vi "RunTest.vi"(8 "error in (no error)":errorcluster, 11 "Prueba06 in":refnum<class "Prueba06.lvclass">) -> (0 "error out":errorcluster, 2 "resultado":string, 3 "Prueba06 out":refnum<class "Prueba06.lvclass">)   [LabVIEW 2019, in "Prueba06.lvclass"]
uses:
  Prueba06.lvclass
  Prueba04/Control/Slide.ctl
  Control/MessageP06.ctl
  Control/EstadosP06.ctl
  Prueba06.lvclass/Prueba06.ctl
  <vilib>/Utility/miscctls.llb/LVRowAndColumnTypeDef.ctl
  ClusterGEN.ctl
  <vilib>/Utility/error.llb/DialogType.ctl
  QMH/Message Queue/Enqueue Message (Single).vi
  <vilib>/Utility/error.llb/Error Cluster From Error Code.vi
  <vilib>/ErrorRing/Error Ring.xnode
  Prueba/Prueba.lvclass
  Prueba04/Prueba04.lvclass
  QMH/User Event - Stop/User Event - Stop.lvlib
  QMH/Message Queue/Message Queue.lvlib
panel:
  out "Message":string
  out "voltaje11":dbl
  out "frecuencia11":dbl
  out "tipoPrueba":string
  out "filaSelecc":i32
  out "TablaVoltajes":string[](array[string])
  out "cumple_no_cumple":bool
  out "n° filas":i32
  out "ptoCentral":dbl=2.0 format="%#.1f"
  out "Vref":dbl
  in  "Tab":enum32{"Page 1", "Page 2"}(tab)
  out "voltaje1":dbl format="%.1f"
  out "RangoRef":string
  out "frecuencia1":dbl=140.0
  in  "guardar_Vref":bool
  out "nivelRef":dbl=95.0 format="%.1f"
  in  "generar1":bool
  in  "AjusteAmp":T1=50.0 caption="Ajuste de amplitud [mV]" scale=0.0..20000.0
  out "frecuencia1":dbl format="%.1f"
  in  "seguir":bool
  out "Pict Ring 3":u16(ring)
  out "Pict Ring 2":u16(ring)
  in  "generar2":bool caption="PruebaSup"
  in  "PruebaInf":bool caption="PruebaSup"
  in  "PruebaSup":bool
  in  "Tabla":string[][](table)
  in  "salir":bool
  out "cumple":bool
  out "no_cumple":bool
  out "voltaje2":dbl format="%.1f"
  out "frecuencia2":dbl format="%.1f"
  in  "cb_rangoRef":string(combo)="1000"
  out "RangoRef2":string
  # "Monitoreo"
  # "Frecuencia"
  # "Elección Señal de Referencia\nsegún marca y modelo de sonómetro"
  # "Hz"
  # "Voltaje"
  # "mV"
  # "Nivel Señal Referencia"
  # "Rango Referencia"
  # "Frecuencia"
  # "6. Linealidad de nivel en el rango de referencia. IEC 61672-3: 2006 Cláusula 14"
  # "Tabla Resultados"
  # "Rango [dBA]"
  # "Referencia [dBA]"
  # "Cumple"
  # "No Cumple"
  # "6. Linealidad de nivel en el rango de referencia. IEC 61672-3: 2006 Cláusula 14"
  # "Monitoreo"
  # "Frecuencia"
  # "Hz"
  # "Voltaje"
  # "mV"
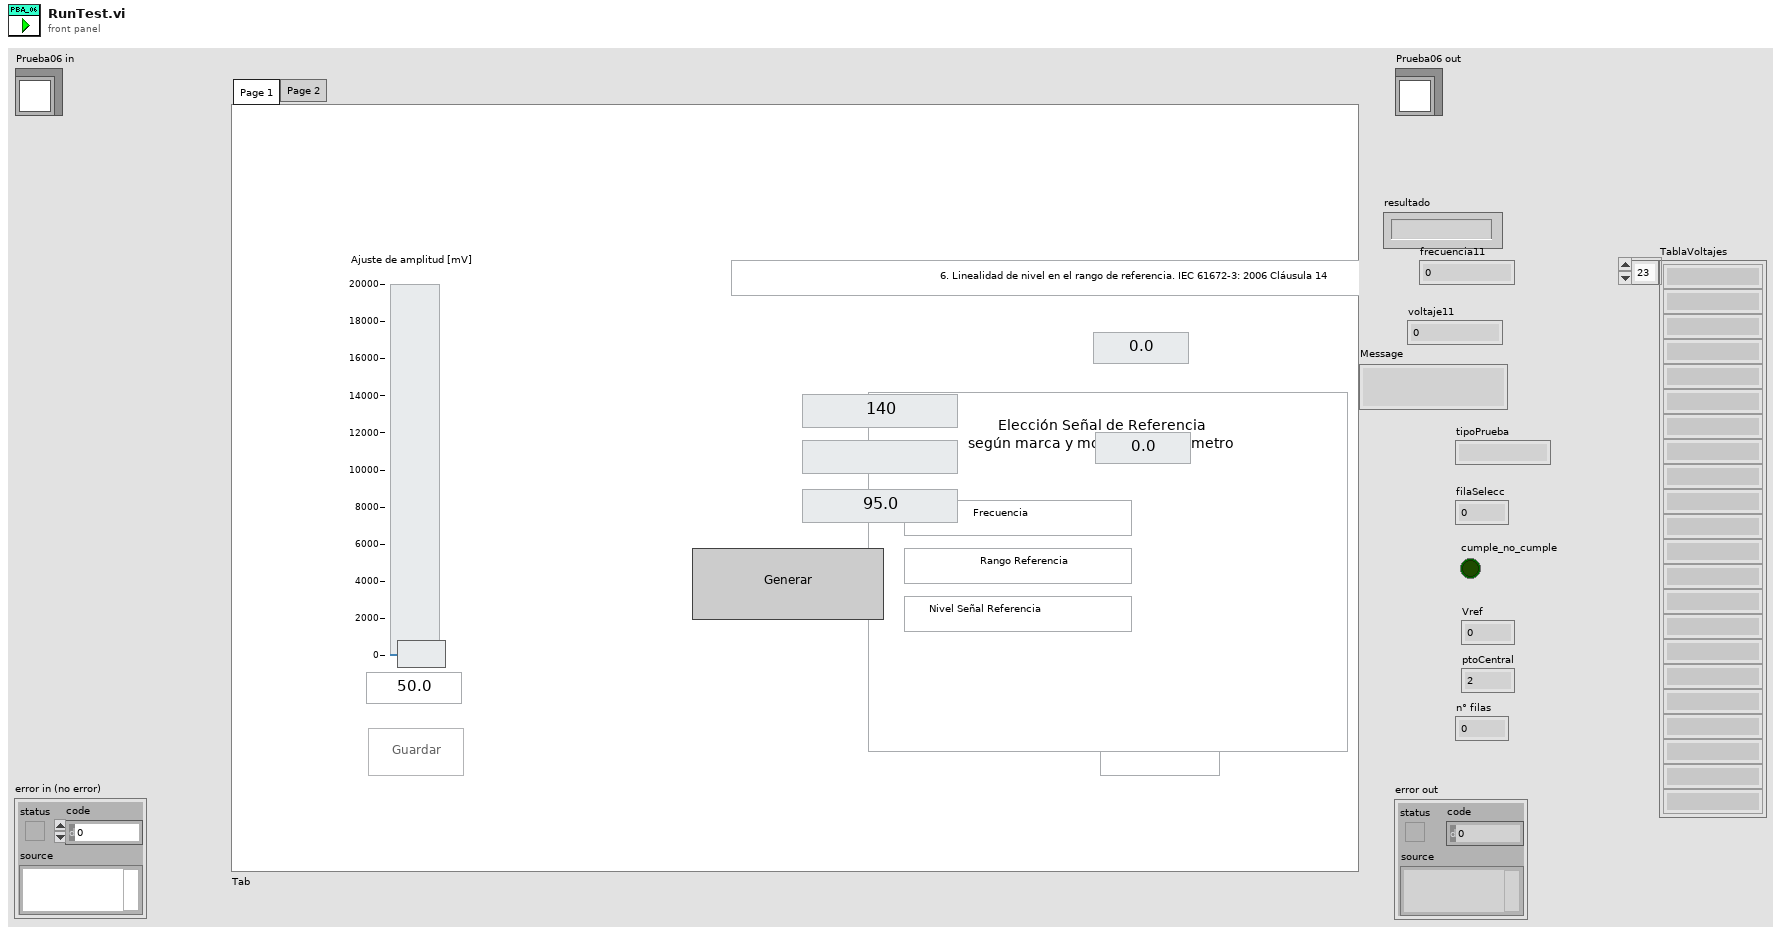
[diagram p1: front panel]
types:
  T1 = typedef "Prueba04.lvclass/Slide.ctl" = dbl
  T2 = typedef "LVRowAndColumnTypeDef.ctl" = cluster{"Row":i32, "Column":i32}
  T3 = typedef "Message Queue.lvlib/All Message Queues.ctl" = cluster{"MHL":refnum<queue>, "Inst_CNT90":refnum<queue>, "Inst_DS360":refnum<queue>, "Inst_Keithley2002":refnum<queue>, "Inst_DAQ":refnum<queue>, "BD":refnum<queue>, "Pistofono":refnum<queue>, "Nexus":refnum<queue>}
  T4 = enum8{"Enabled", "Disabled", "Disabled and Grayed Out"}
  T5 = typedef "Prueba06.lvclass/MessageP06.ctl" = cluster{"Estado":T6, "Data":variant}
  T6 = typedef "Prueba06.lvclass/EstadosP06.ctl" = enum16{"inicio", "LeerArchivoConfiguracion", "ConfirmarSalida", "DetieneInstrumentos", "InicializaInstrumento", "leerRango", "configuraRango", "calcularVref", "configuraTabla", "FrecAmp1", "FrecAmp2", "iniciarGEN", "monitoreo", "detenerGEN", "ajusteAmp", "guardaVerf", "creaVoltPrueba", "preguntaTipoPrueba", "guardarMediciones", "ingresaMediciones", "cumplimiento", "listo_evaluar", "evaluar", "final", "salir"}
  T7 = enum32{"Page 1", "Page 2", "Page 3", "Page 4", "Page 5", "Page 6", "Page 7"}
  T8 = typedef "Prueba06.lvclass/ClusterGEN.ctl" = cluster{"frec":dbl, "amp":dbl}
  T9 = cluster{"ControlName":string, "ControlReference":refnum<vi>}[]
  T10 = typedef "DialogType.ctl" = u16
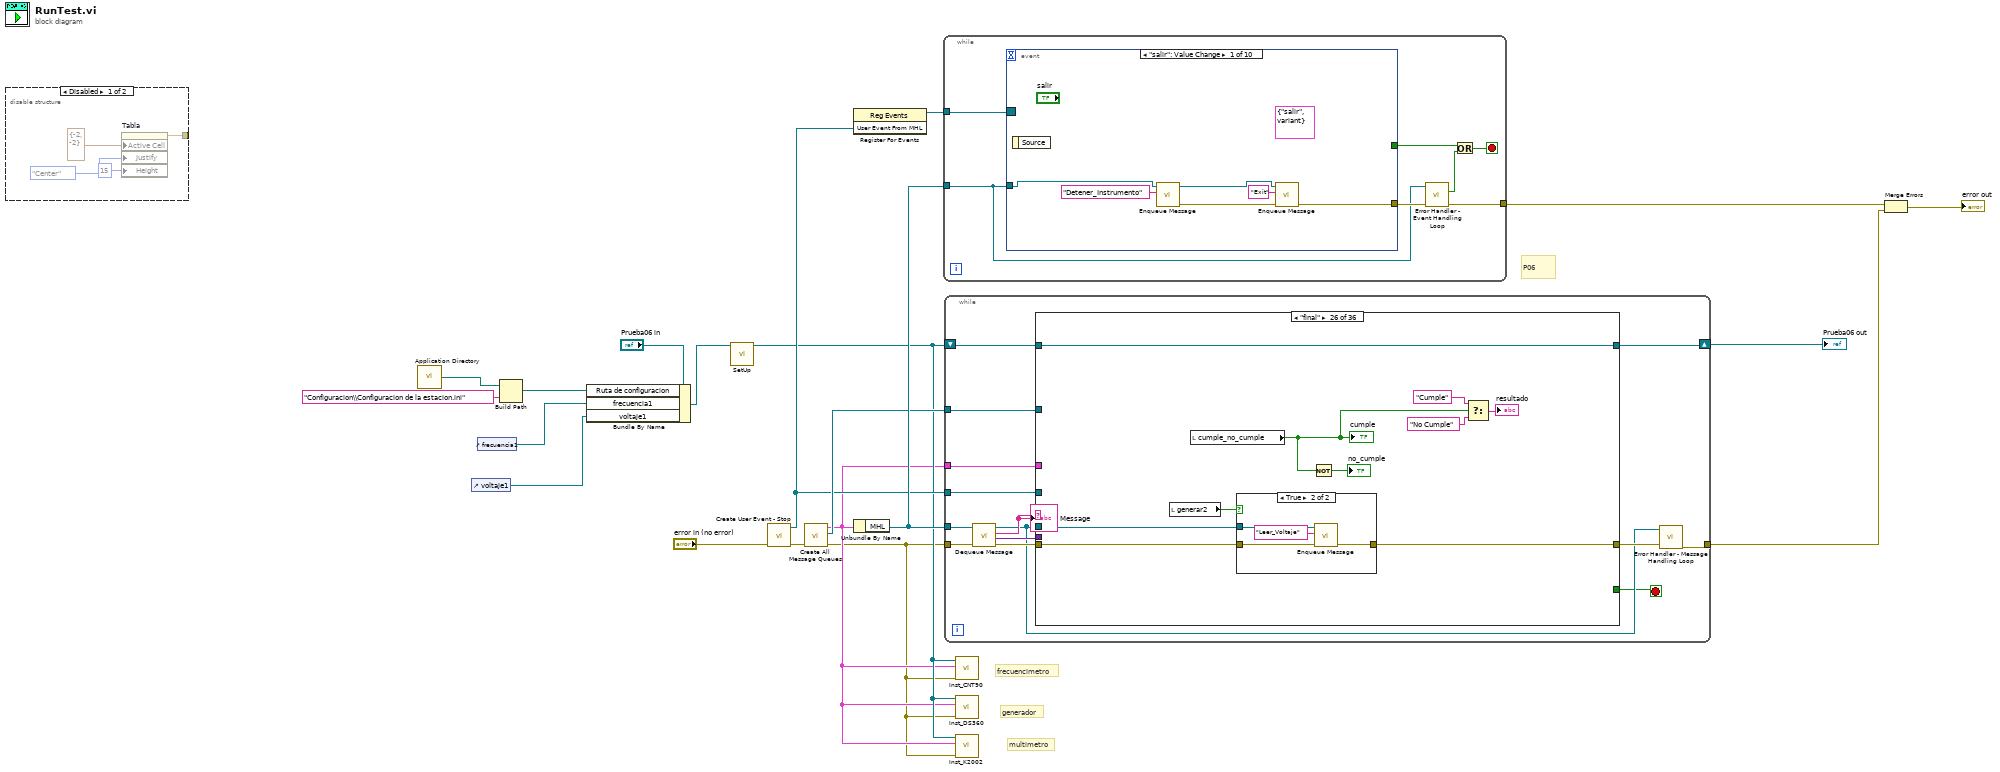
[diagram p0: block diagram]
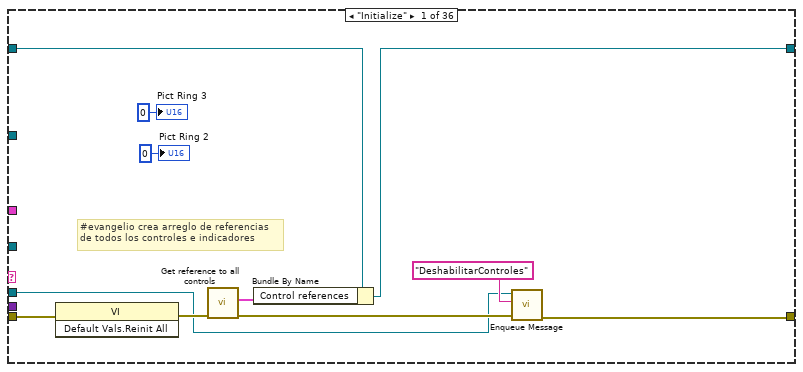
[diagram p3: hidden frame]
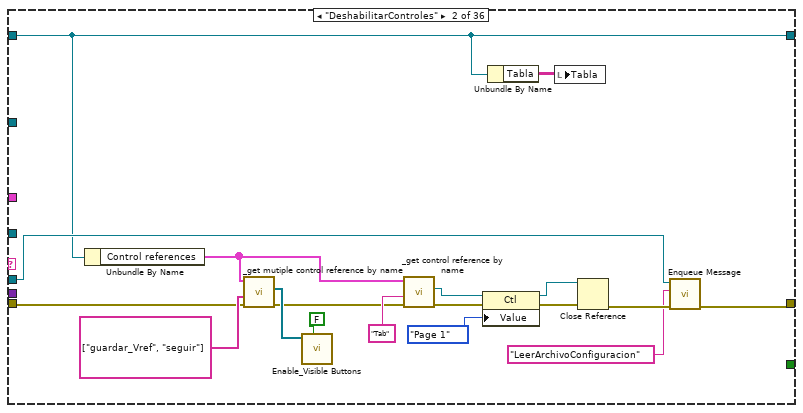
[diagram p4: hidden frame]
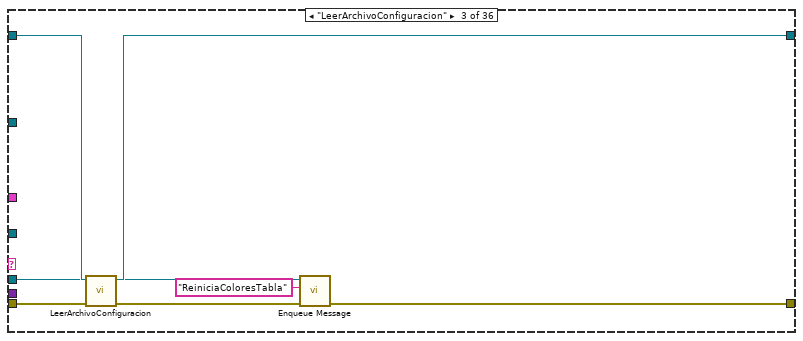
[diagram p5: hidden frame]
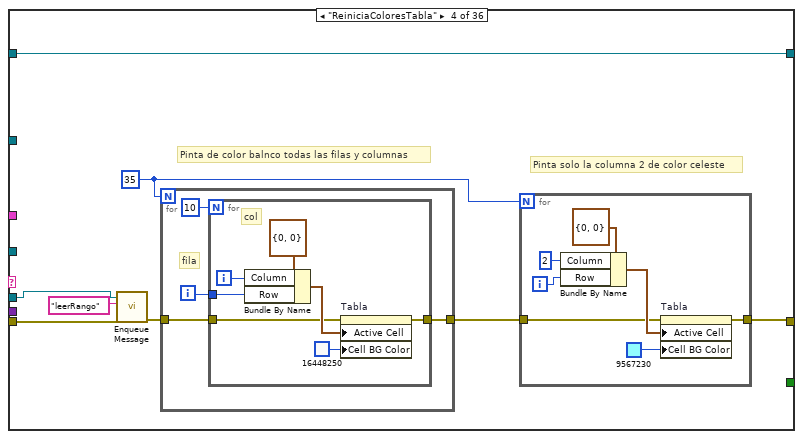
[diagram p6: hidden frame]
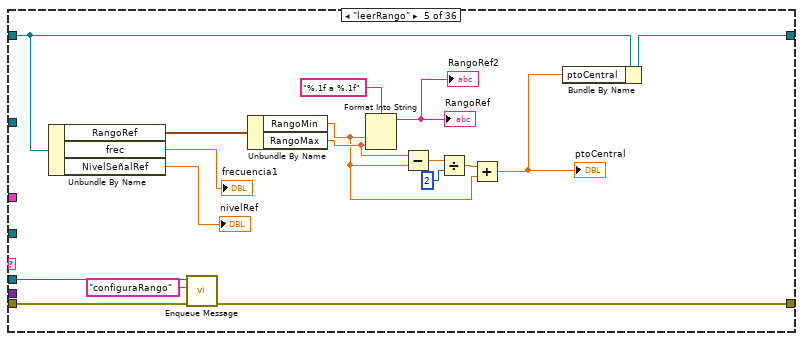
[diagram p7: hidden frame]
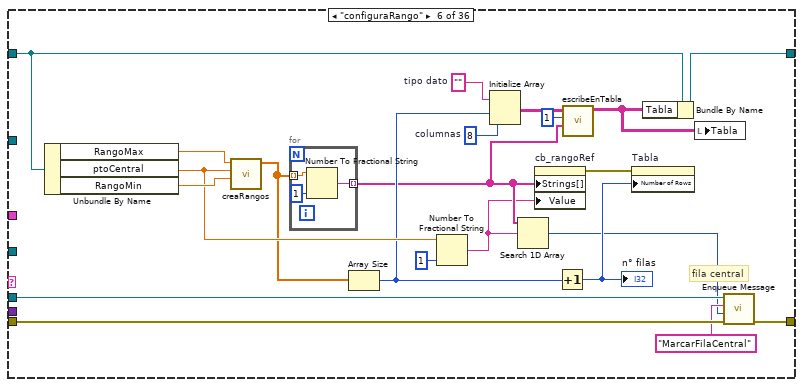
[diagram p8: hidden frame]
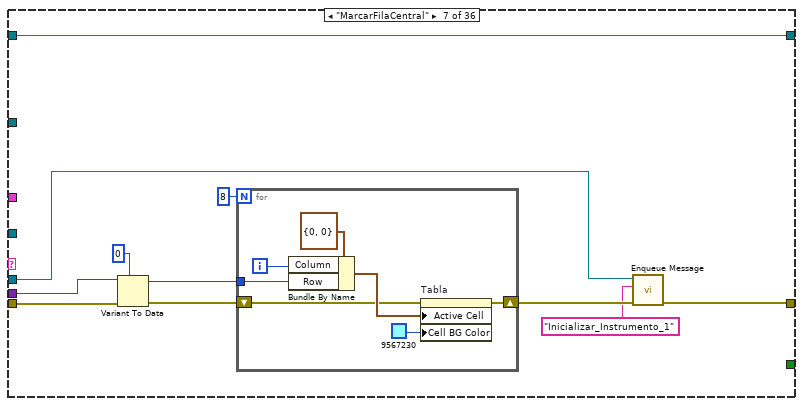
[diagram p9: hidden frame]
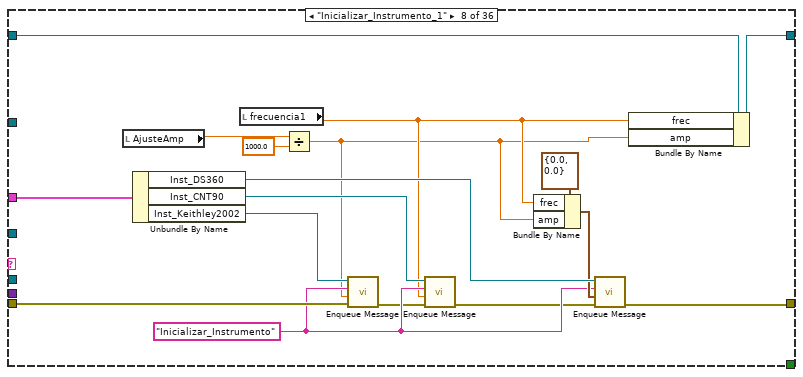
[diagram p10: hidden frame]
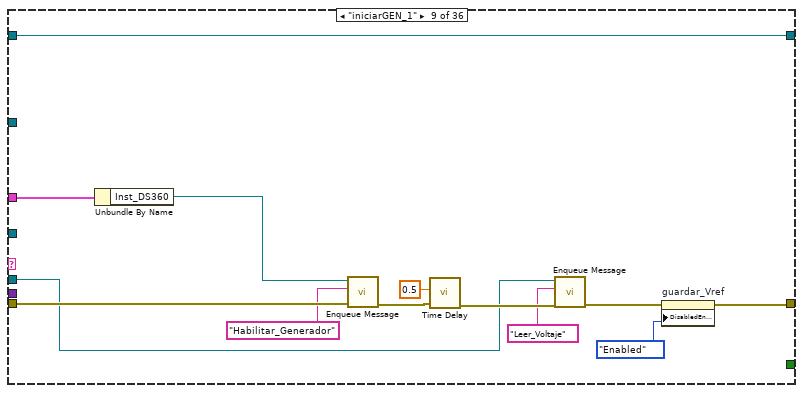
[diagram p11: hidden frame]
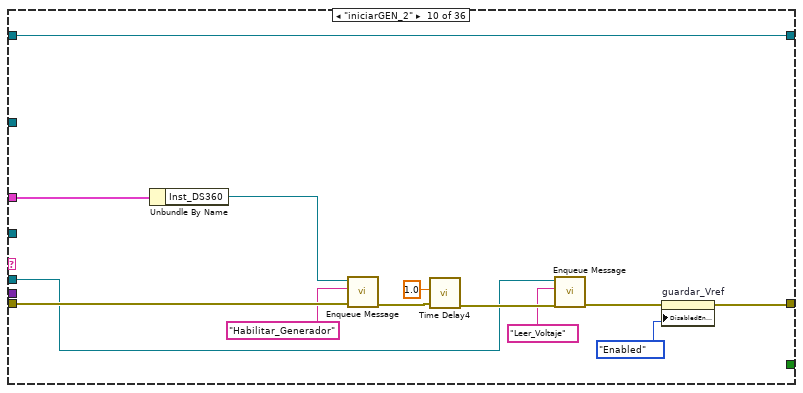
[diagram p12: hidden frame]
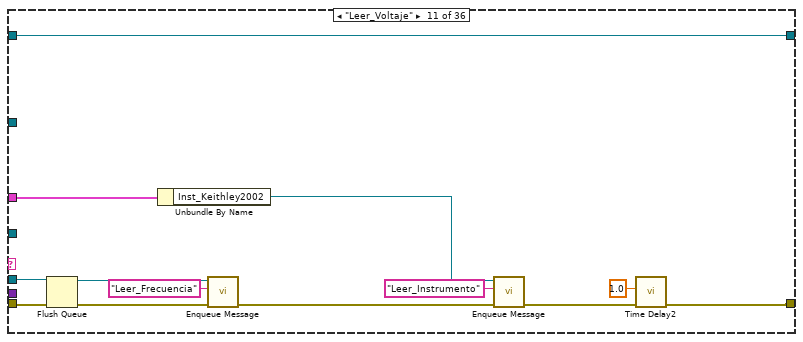
[diagram p13: hidden frame]
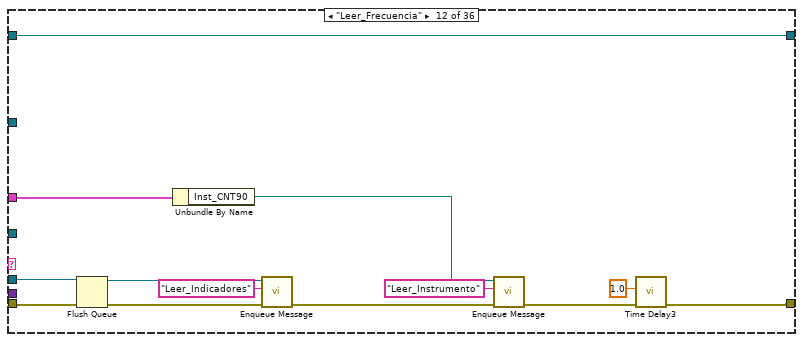
[diagram p14: hidden frame]
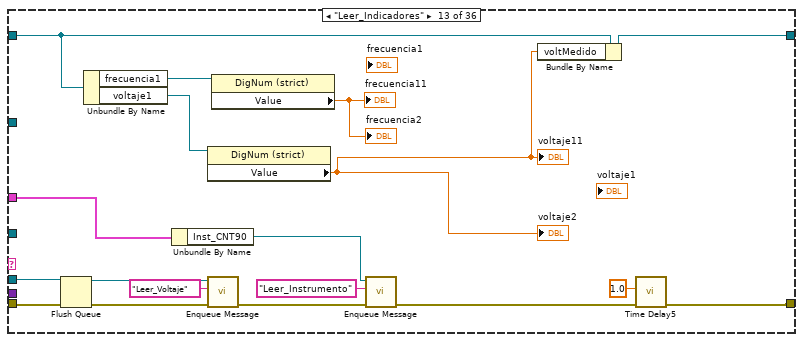
[diagram p15: hidden frame]
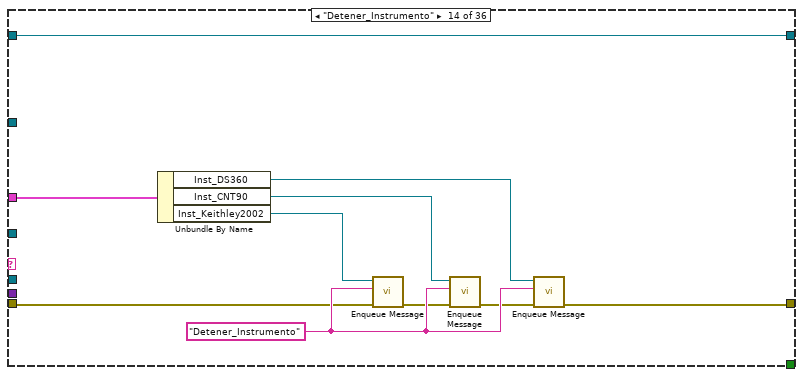
[diagram p16: hidden frame]
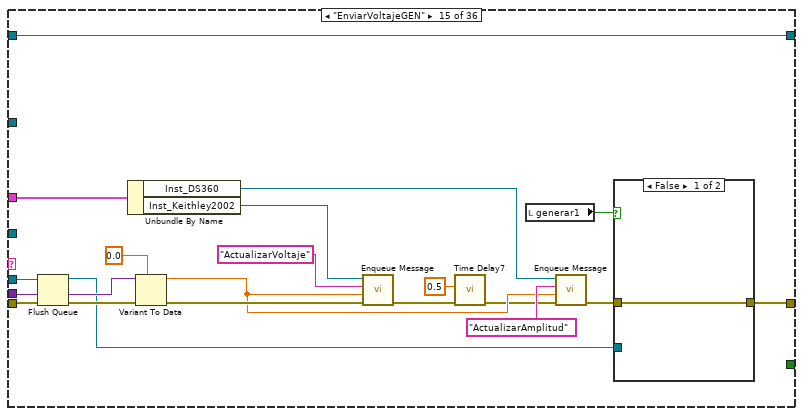
[diagram p17: hidden frame]
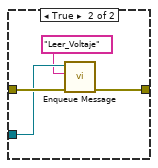
[diagram p18: hidden frame]
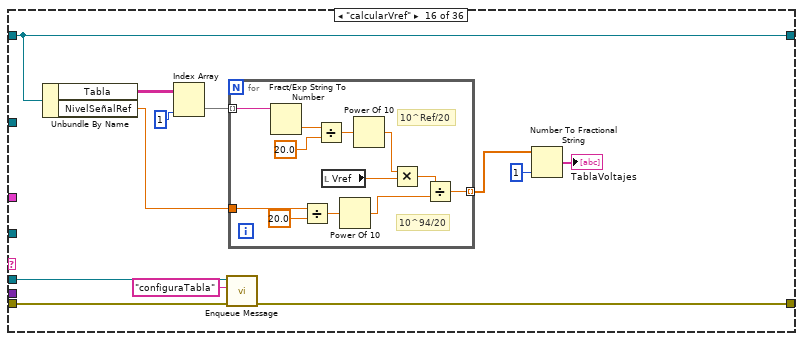
[diagram p19: hidden frame]
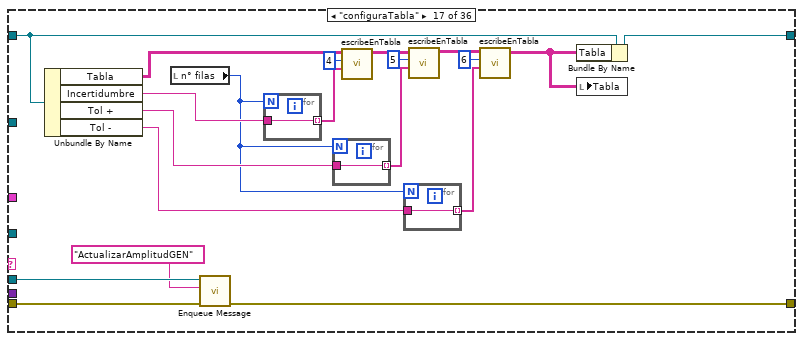
[diagram p20: hidden frame]
diagram:
  # "P06"
  # "multimetro"
  # "generador"
  # "frecuencimetro"
  n1 = disable-structure shown="Disabled" {
    disable-tunnel: [w23 _] -> _
    frame Disabled {
      n2 = property on="Tabla" class="Tbl (strict)"("Active Cell"=T2 {"Row"=-2, "Column"=-2} ("Active Cell:Active Cell"), "Justify"=enum16{"Left", "Center", "Right"}."Center" ("Active Cell:Cell Justification"), "Height"=u32 15 ("Active Cell:Cell Font:Size")) -> (error out=w23:errorcluster)  [unwired: 2 in, 1 out]
    }
    frame Enabled {
    }
  }
  n3 = call <vilib>:"Application Directory.vi"() -> ("Application Directory"=w15:path)
  n4 = control-ref of="voltaje1"() -> (w1:refnum<vi>)
  n5 = control-ref of="frecuencia1"() -> (w2:refnum<vi>)
  n6 = Build Path(base path=w15, name or relative path="Configuracion\\Configuracion de la estacion.ini") -> (appended path=w14:path)
  n7 = Bundle By Name(cluster="Prueba06 in", "Ruta de configuracion"=w14, "frecuencia1"=w2, "voltaje1"=w1) -> (w12:refnum<class "Prueba06.lvclass">)
  n8 = call-dynamic "SetUp.vi"("Prueba06 in"=w12) -> ("Prueba06 out"=w5:refnum<class "Prueba06.lvclass">)  [unwired: 9 in, 1 out]
  n9 = call "Create User Event - Stop.vi"("error in (no error)"="error in (no error)") -> ("error out"=w11:errorcluster, "User Event From MHL"=w7:refnum<user-event>)  [unwired: 9 in]
  n10 = call "Create All Message Queues.vi"("error in (no error)"=w11) -> ("error out"=w3:errorcluster, "PL Queues Array"=w8:refnum<queue>[], "All Message Queues out"=w4:T3)  [unwired: 8 in]
  n11 = register-events(w7) -> (reference out=w6:refnum<event-registration>)  [unwired: 2 in, 1 out]
  n12 = Unbundle By Name(w4) -> ("MHL"=w9:refnum<queue>)
  n13 = while {
    tunnel: w9 -> [w25]
    tunnel: [w29] -> w19
    tunnel: w6 -> [w27]
    stop <- w28 stop-if-true
    n14 = event shown="[0] \"salir\": Value Change" {
      selector: w27 -> [_ _ _ _ _ _ _ _ _ _]
      dyn-events: _ -> [_ _ _ _ _ _ _ _ _ _]
      timeout: _ -> [_ _ _ _ _ _ _ _ _ _]
      tunnel: w25 -> [w34 _ w45 w53 w60 w72 w78 w83 w88 w92]
      tunnel: [w37 _ _ w48 w55 w68 w79 w81 w87 w91] -> w30
      tunnel: [_ w38 _ _ _ _ _ _ _ _] -> w26
      event "salir": Value Change {
        (unwired) T5 {"Estado"=enum."salir", "Data"=variant} ("element")
        n15 = event-data() -> ()  [unwired: 1 in, 1 out]
        n16 = call-poly "Enqueue Message.vi"("Message"="Detener_Instrumento", "Message Queue"=w34) -> ("error out"=w32:errorcluster, "dup Message Queue"=w33:refnum<queue>)  [unwired: 8 in]
        n17 = call-poly "Enqueue Message.vi"("error in (no error)"=w32, "Message"="Exit", "Message Queue"=w33) -> ("error out"=w37:errorcluster)  [unwired: 7 in, 1 out]
      }
      event User Event {
        n18 = event-data() -> ("User Event"=w40:string, "Event Data"=w39:variant)  [unwired: 1 in]
        n19 = case shown="\"Exit EHL\"" w40 {
          tunnel: w39 -> [_ w42]
          tunnel: [_ w41] -> w38
          frame Default {
          }
          frame "Exit EHL" {
            # "#evangelio Termina\nla ejecucion del EHL"
            n20 = Variant To Data(type=TRUE, Variant=w42) -> (data=w41:bool)  [unwired: 1 in, 1 out]
          }
        }
      }
      event Panel Close? {
        w44 = TRUE
        n21 = event-data() -> ()  [unwired: 1 in, 1 out]
        n22 = call-poly "Enqueue Message.vi"("Priority Message? (F)"=w44, "Message"="Confirmar Salida", "Message Queue"=w45) -> ()  [unwired: 7 in, 2 out]
        n23 = event-data("Discard?"=w44) -> ()  [unwired: 1 in, 1 out]
      }
      event "generar1": Value Change {
        n24 = event-data() -> ("NewVal"=w52:bool)  [unwired: 1 in]
        n25 = Select(t="iniciarGEN_1", s=w52, f="detenerGEN") -> (s? t:f=w49:string)
        n26 = call-poly "Enqueue Message.vi"("Priority Message? (F)"=TRUE, "Message"=w49, "Message Queue"=w53) -> ("error out"=w48:errorcluster)  [unwired: 7 in, 1 out]
      }
      event "generar2": Value Change {
        n27 = event-data() -> ("NewVal"=w59:bool)  [unwired: 1 in]
        n28 = Select(t="preguntaTipoPrueba", s=w59, f="guardarMediciones") -> (s? t:f=w54:string)
        n29 = call-poly "Enqueue Message.vi"("Priority Message? (F)"=TRUE, "Message"=w54, "Message Queue"=w60) -> ("error out"=w61:errorcluster)  [unwired: 7 in, 1 out]
        n30 = case shown="\"preguntaTipoPrueba\", Default" w54 {
          tunnel: w61 -> [w64 w67]
          tunnel: [w63 w66] -> w55
          frame "preguntaTipoPrueba", Default {
            n31 = property on="cb_rangoRef" class="CmbBox"(error in=w64, "DisabledEnum"=T4."Disabled" ("Disabled")) -> (error out=w63:errorcluster)  [unwired: 1 in, 1 out]
          }
          frame "guardarMediciones" {
            n32 = property on="cb_rangoRef" class="CmbBox"(error in=w67, "DisabledEnum"=T4."Enabled" ("Disabled")) -> (error out=w66:errorcluster)  [unwired: 1 in, 1 out]
          }
        }
      }
      event "seguir": Value Change {
        n33 = event-data() -> ()  [unwired: 1 in, 1 out]
        n34 = call-poly "Enqueue Message.vi"("Message"="calcularVref", "Message Queue"=w72) -> ("error out"=w69:errorcluster)  [unwired: 8 in, 1 out]
        n35 = property on="Tab" class="TabCtl (strict)"(error in=w69, "Value"=enum32{"Page 1", "Page 2"}."Page 2" ("Tab")) -> (error out=w68:errorcluster)  [unwired: 1 in, 1 out]
      }
      event Value Change {
        (unwired) T5 {"Estado"=enum."FrecAmp1", "Data"=variant} ("element")
        n36 = event-data() -> ()  [unwired: 1 in, 1 out]
        n37 = Divide(x="AjusteAmp", y=T1 1000.0) -> (x/y=w74:T1)
        n38 = call-poly "Enqueue Message.vi"("Priority Message? (F)"=TRUE, "Message Data"=w74, "Message"="EnviarVoltajeGEN", "Message Queue"=w78) -> ("error out"=w79:errorcluster)  [unwired: 6 in, 1 out]
      }
      event "guardar_Vref": Value Change {
        (unwired) T5 {"Estado"=enum."guardaVerf", "Data"=variant} ("element")
        n39 = event-data() -> ()  [unwired: 1 in, 1 out]
        n40 = call-poly "Enqueue Message.vi"("Priority Message? (F)"=TRUE, "Message"="guardaVerf", "Message Queue"=w83) -> ("error out"=w81:errorcluster)  [unwired: 7 in, 1 out]
      }
      event "Tabla": Value Change {
        n41 = event-data() -> ("NewVal"=w85:string[][])  [unwired: 1 in]
        n42 = call-poly "Enqueue Message.vi"("Priority Message? (F)"=TRUE, "Message Data"=w85, "Message"="ingresaMediciones", "Message Queue"=w88) -> ("error out"=w87:errorcluster)  [unwired: 6 in, 1 out]
      }
      event "cb_rangoRef": Value Change {
        n43 = event-data() -> ()  [unwired: 1 in, 1 out]
        n44 = call-poly "Enqueue Message.vi"("Priority Message? (F)"=TRUE, "Message"="ActualizarAmplitudGEN", "Message Queue"=w92) -> ("error out"=w91:errorcluster)  [unwired: 7 in, 1 out]
      }
    }
    n45 = call "Error Handler - Event Handling Loop.vi"("error in (no error)"=w30, "Message Queue"=w25) -> ("dup error in"=w29:errorcluster, "Error?"=w31:bool)  [unwired: 7 in, 1 out]
    n46 = Or(x=w26, y=w31) -> (x .or. y?=w28:bool)
  }
  n47 = while {
    tunnel: w9 -> [w104]
    tunnel: w3 -> [w103]
    tunnel: [w93] -> w18
    shift-right: [w105] -> w20
    shift-left: w5 -> [w106]
    tunnel: w4 -> [w98]
    tunnel: w8 -> [w97]
    tunnel: w7 -> [w99]
    stop <- w94 stop-if-true
    n48 = call "Dequeue Message.vi"("error in (no error)"=w103, "Message Queue"=w104) -> ("error out"=w102:errorcluster, "Message Data"=w100:variant, "Message"=w101:string, "dup Message Queue"=w95:refnum<queue>)  [unwired: 6 in]
    "Message" <- w101
    n49 = case shown="\"final\"" w101 {
      selector: w101 -> [_ _ _ _ _ _ _ _ _ _ _ _ _ _ _ _ _ _ _ _ _ _ _ _ _ _ _ _ _ _ _ w639 _ _ _ w677]
      tunnel: [w110 w119 w140 w150 w184 w203 w221 w244 w258 w271 w284 w297 w300 w316 w345 w360 w387 w417 w442 w452 w465 w495 w510 w518 w543 w564 w574 w576 w590 w609 w623 w630 w655 w673 w675 w678] -> w105
      tunnel: w106 -> [w111 w119 w141 w150 w185 w205 w221 w245 w258 w271 w284 w297 w306 w316 w345 w360 w388 w418 w443 w452 w482 w506 w514 w518 w543 w564 w574 w581 w590 w609 w623 w631 w655 w673 w675 w678]
      tunnel: w100 -> [_ _ _ _ _ _ w219 _ _ _ _ _ _ _ w335 _ _ _ _ _ _ w499 _ _ _ _ w572 w578 _ _ _ _ _ w664 _ _]
      tunnel: w102 -> [w112 w121 w142 w148 w183 w197 w220 w243 w257 w270 w276 w289 w308 w319 w336 w358 w386 w416 w441 w448 w483 w508 w516 w525 w546 w562 w573 w580 w592 w611 w622 w640 w650 w667 w674 _]
      tunnel: [w109 w118 w137 w144 w174 w191 w213 w233 w253 w266 w275 w288 w307 w317 w328 w356 w377 w402 w433 w445 w462 w505 w513 w524 w544 w557 w571 w579 w591 w610 w619 w635 w648 w665 w674 w676] -> w96
      tunnel: [_ _ _ _ _ _ _ _ _ _ _ _ _ _ _ _ _ _ _ _ _ _ _ _ _ _ _ _ _ _ _ w636 _ _ _ _] -> w94
      tunnel: w95 -> [w113 w120 w138 w147 w173 w190 w212 _ w247 w260 w273 w286 w302 _ w331 w357 w376 _ _ w446 w479 w502 w512 w523 w545 w556 _ _ w583 w603 _ w634 w649 w666 _ _]
      tunnel: w99 -> [_ _ _ _ _ _ _ _ _ _ _ _ _ _ _ _ _ _ _ _ _ _ _ _ _ _ _ _ _ _ _ w637 _ _ _ _]
      tunnel: w98 -> [_ _ _ _ _ _ _ w229 w252 w265 w277 w290 w309 w318 w334 _ _ w401 w432 _ _ _ _ _ _ _ _ _ w593 w612 _ _ _ _ _ _]
      tunnel: w97 -> [_ _ _ _ _ _ _ _ _ _ _ _ _ _ _ _ _ _ _ _ _ _ _ _ _ _ _ _ _ _ _ w638 _ _ _ _]
      frame "Initialize" {
        # "#evangelio crea arreglo de referencias\nde todos los controles e indicadores"
        n50 = invoke class="VI" method="Default Vals.Reinit All"(error in=w112) -> (error out=w116:errorcluster)  [unwired: 2 in, 2 out]
        n51 = call "Get reference to all controls.vi"("error in (no error)"=w116) -> ("error out"=w114:errorcluster, "Control references"=w115:T9)  [unwired: 5 in]
        n52 = Bundle By Name(cluster=w111, "Control references"=w115) -> (w110:refnum<class "Prueba06.lvclass">)
        n53 = call-poly "Enqueue Message.vi"("error in (no error)"=w114, "Message"="DeshabilitarControles", "Message Queue"=w113) -> ("error out"=w109:errorcluster)  [unwired: 7 in, 1 out]
        "Pict Ring 2" <- u16 0 ("Pict Ring 2")
        "Pict Ring 3" <- u16 0 ("Pict Ring 3")
      }
      frame "DeshabilitarControles" {
        n54 = Unbundle By Name(w119) -> ("Control references"=w130:T9)
        n55 = call "_get mutiple control reference by name.vi"("error in (no error)"=w121, "Control names"=string[] ["guardar_Vref", "seguir"], "Control references"=w130) -> ("error out"=w127:errorcluster, "References"=w128:refnum<vi>[])  [unwired: 3 in]
        n56 = call "Enable_Visible Buttons.vi"("Enable? (T)"=FALSE, "Controls Ref Array"=w128) -> ()  [unwired: 10 in]
        n57 = call "_get control reference by name.vi"("error in (no error)"=w127, "Control name"="Tab" ("Message"), "Control references"=w130) -> ("error out"=w134:errorcluster, "Ctl Refnum"=w132:refnum<vi>)  [unwired: 3 in]
        n58 = property class="Ctl"(reference=w132, error in=w134, "Value"=T7."Page 1" ("Tab_Prueba04")) -> (reference out=w123:refnum<vi>, error out=w125:errorcluster)
        n59 = Unbundle By Name(w119) -> ("Tabla"=w135:string[][])
        n60 = local write "Tabla"(w135) -> ()
        n61 = Close Reference(reference=w123, error in (no error)=w125) -> (error out=w124:errorcluster)
        n62 = call-poly "Enqueue Message.vi"("error in (no error)"=w124, "Message"="LeerArchivoConfiguracion", "Message Queue"=w120) -> ("error out"=w118:errorcluster)  [unwired: 7 in, 1 out]
      }
      frame "LeerArchivoConfiguracion" {
        n63 = call "LeerArchivoConfiguracion.vi"("error in"=w142, "Prueba06 in"=w141) -> ("error out"=w139:errorcluster, "Prueba06 out"=w140:refnum<class "Prueba06.lvclass">)  [unwired: 8 in]
        n64 = call-poly "Enqueue Message.vi"("error in (no error)"=w139, "Message"="ReiniciaColoresTabla", "Message Queue"=w138) -> ("error out"=w137:errorcluster)  [unwired: 7 in, 1 out]
      }
      frame "ReiniciaColoresTabla" {
        w143 = 35
        # "Pinta solo la columna 2 de color celeste"
        # "Pinta de color balnco todas las filas y columnas"
        n65 = call-poly "Enqueue Message.vi"("error in (no error)"=w148, "Message"="leerRango", "Message Queue"=w147) -> ("error out"=w146:errorcluster)  [unwired: 7 in, 1 out]
        n66 = for {
          N: w143 -> [_]
          tunnel: w146 -> [w154]
          tunnel: [w153] -> w145
          i -> [w152]
          # "fila"
          n67 = for {
            N: 10 -> [_]
            tunnel: [w158] -> w153
            tunnel: w154 -> [w157]
            tunnel: w152 -> [w156]
            i -> [w155]
            # "col"
            n68 = Bundle By Name(cluster=T2 {"Row"=0, "Column"=0} ("Active Cell:Active Cell"), "Column"=w155, "Row"=w156) -> (w160:T2)
            n69 = property on="Tabla" class="Tbl (strict)"(error in=w157, "Active Cell"=w160, "Cell BG Color"=u32 16448250) -> (error out=w158:errorcluster)  [unwired: 1 in, 1 out]
          }
        }
        n70 = for {
          N: w143 -> [_]
          tunnel: [w164] -> w144
          tunnel: w145 -> [w162]
          i -> [w163]
          n71 = Bundle By Name(cluster=T2 {"Row"=0, "Column"=0} ("Active Cell:Active Cell"), "Column"=2, "Row"=w163) -> (w166:T2)
          n72 = property on="Tabla" class="Tbl (strict)"(error in=w162, "Active Cell"=w166, "Cell BG Color"=u32 9567230) -> (error out=w164:errorcluster)  [unwired: 1 in, 1 out]
        }
      }
      frame "leerRango" {
        n73 = Unbundle By Name(w185) -> ("RangoRef"=w182:cluster{"RangoMin":dbl, "RangoMax":dbl}, "frec"=→"frecuencia1":dbl, "NivelSeñalRef"=→"nivelRef":dbl)
        n74 = call-poly "Enqueue Message.vi"("error in (no error)"=w183, "Message"="configuraRango", "Message Queue"=w173) -> ("error out"=w174:errorcluster)  [unwired: 7 in, 1 out]
        n75 = Unbundle By Name(w182) -> ("RangoMin"=w175:dbl, "RangoMax"=w180:dbl)
        n76 = Format Into String(format string="%.1f a %.1f", w175, w180) -> (resulting string=→"RangoRef" →"RangoRef2":string)  [unwired: 2 in, 1 out]
        n77 = Subtract(x=w180, y=w175) -> (x-y=w177:dbl)
        n78 = Divide(x=w177, y=u32 2) -> (x/y=w178:dbl)
        n79 = Add(x=w178, y=w175) -> (x+y=w179:dbl)
        "ptoCentral" <- w179
        n80 = Bundle By Name(cluster=w185, "ptoCentral"=w179) -> (w184:refnum<class "Prueba06.lvclass">)
      }
      frame "configuraRango" {
        w196 = 8  # columnas
        w195 = ""  # tipo dato
        # "fila central"
        n81 = Unbundle By Name(w205) -> ("RangoMax"=w207:dbl, "ptoCentral"=w202:dbl, "RangoMin"=w206:dbl)
        n82 = call "creaRangos.vi"("RangoMin"=w206, "ptoCentral"=w202, "RangoMax"=w207) -> ("RangoCompleto"=w201:dbl[])  [unwired: 5 in, 3 out]
        n83 = for {
          tunnel: w201 -> [w210] mode=indexing
          tunnel: [w209] -> w188 mode=indexing
          n84 = Number To Fractional String(number=w210, precision (6)=i16 1) -> (F-format string=w209:string)  [unwired: 2 in]
        }
        n85 = Array Size(array=w201) -> (size(s)=w194:i32)
        n86 = Number To Fractional String(number=w202, precision (6)=i16 1) -> (F-format string=w187:string)  [unwired: 2 in]
        n87 = Initialize Array(w195, w194, w196) -> (w193:string[][])
        n88 = Search 1D Array(1D array=w188, element=w187) -> (index of element=w186:i32)  [unwired: 1 in]
        n89 = property on="cb_rangoRef" class="CmbBox"("Strings[]"=w188, "Value"=w187) -> (error out=w200:errorcluster)  [unwired: 2 in, 1 out]
        n90 = Increment(x=w194) -> (x+1=w199:i32)
        "n° filas" <- w199
        n91 = call "escribeEnTabla.vi"("parametros"=w188, "col"=1, "tabla in"=w193) -> ("tabla out"=w192:string[][])  [unwired: 8 in]
        n92 = property on="Tabla" class="Tbl (strict)"(error in=w200, "Number of Rows"=w199) -> ()  [unwired: 1 in, 2 out]
        n93 = Bundle By Name(cluster=w205, "Tabla"=w192) -> (w203:refnum<class "Prueba06.lvclass">)
        n94 = local write "Tabla"(w192) -> ()
        n95 = call-poly "Enqueue Message.vi"("error in (no error)"=w197, "Message Data"=w186, "Message"="MarcarFilaCentral", "Message Queue"=w190) -> ("error out"=w191:errorcluster)  [unwired: 6 in, 1 out]
      }
      frame "MarcarFilaCentral" {
        n96 = Variant To Data(error in=w220, type=0, Variant=w219) -> (data=w215:i32, error out=w217:errorcluster)
        n97 = for {
          N: 8 -> [_]
          tunnel: w215 -> [w223]
          shift-right: [w224] -> w216
          shift-left: w217 -> [w225]
          i -> [w222]
          n98 = Bundle By Name(cluster=T2 {"Row"=0, "Column"=0} ("Active Cell:Active Cell"), "Column"=w222, "Row"=w223) -> (w227:T2)
          n99 = property on="Tabla" class="Tbl (strict)"(error in=w225, "Active Cell"=w227, "Cell BG Color"=u32 9567230) -> (error out=w224:errorcluster)  [unwired: 1 in, 1 out]
        }
        n100 = call-poly "Enqueue Message.vi"("error in (no error)"=w216, "Message"="Inicializar_Instrumento_1", "Message Queue"=w212) -> ("error out"=w213:errorcluster)  [unwired: 7 in, 1 out]
      }
      frame "Inicializar_Instrumento_1" {
        w236 = "Inicializar_Instrumento" ("Message")
        n101 = local read "AjusteAmp"() -> (w242:T1)
        n102 = Unbundle By Name(w229) -> ("Inst_DS360"=w240:refnum<queue>, "Inst_CNT90"=w239:refnum<queue>, "Inst_Keithley2002"=w238:refnum<queue>)
        n103 = local read "frecuencia1"() -> (w231:dbl)
        n104 = Divide(x=w242, y=T1 1000.0) -> (x/y=w230:T1)
        n105 = call-poly "Enqueue Message.vi"("error in (no error)"=w243, "Message Data"=w230, "Message"=w236, "Message Queue"=w238) -> ("error out"=w235:errorcluster)  [unwired: 6 in, 1 out]
        n106 = call-poly "Enqueue Message.vi"("error in (no error)"=w235, "Message Data"=w231, "Message"=w236, "Message Queue"=w239) -> ("error out"=w234:errorcluster)  [unwired: 6 in, 1 out]
        n107 = Bundle By Name(cluster=T8 {"frec"=0.0, "amp"=0.0} ("clusterGEN"), "frec"=w231, "amp"=w230) -> (w237:T8)
        n108 = call-poly "Enqueue Message.vi"("error in (no error)"=w234, "Message Data"=w237, "Message"=w236, "Message Queue"=w240) -> ("error out"=w233:errorcluster)  [unwired: 6 in, 1 out]
        n109 = Bundle By Name(cluster=w245, "frec"=w231, "amp"=w230) -> (w244:refnum<class "Prueba06.lvclass">)
      }
      frame "iniciarGEN_1" {
        n110 = Unbundle By Name(w252) -> ("Inst_DS360"=w251:refnum<queue>)
        n111 = call-poly "Enqueue Message.vi"("error in (no error)"=w257, "Message"="Habilitar_Generador", "Message Queue"=w251) -> ("error out"=w249:errorcluster)  [unwired: 7 in, 1 out]
        n112 = call "Time Delay"("error in (no error)"=w249, "Delay Time (s)"=0.5) -> ("error out"=w248:errorcluster)  [unwired: 9 in]
        n113 = call-poly "Enqueue Message.vi"("error in (no error)"=w248, "Message"="Leer_Voltaje", "Message Queue"=w247) -> ("error out"=w254:errorcluster)  [unwired: 7 in, 1 out]
        n114 = property on="guardar_Vref" class="Bool"(error in=w254, "DisabledEnum"=T4."Enabled" ("Disabled")) -> (error out=w253:errorcluster)  [unwired: 1 in, 1 out]
      }
      frame "iniciarGEN_2" {
        n115 = Unbundle By Name(w265) -> ("Inst_DS360"=w264:refnum<queue>)
        n116 = call-poly "Enqueue Message.vi"("error in (no error)"=w270, "Message"="Habilitar_Generador", "Message Queue"=w264) -> ("error out"=w262:errorcluster)  [unwired: 7 in, 1 out]
        n117 = call "Time Delay4"("error in (no error)"=w262, "Delay Time (s)"=1.0) -> ("error out"=w261:errorcluster)  [unwired: 9 in]
        n118 = call-poly "Enqueue Message.vi"("error in (no error)"=w261, "Message"="Leer_Voltaje", "Message Queue"=w260) -> ("error out"=w267:errorcluster)  [unwired: 7 in, 1 out]
        n119 = property on="guardar_Vref" class="Bool"(error in=w267, "DisabledEnum"=T4."Enabled" ("Disabled")) -> (error out=w266:errorcluster)  [unwired: 1 in, 1 out]
      }
      frame "Leer_Voltaje" {
        n120 = Flush Queue(queue=w273, error in (no error)=w276) -> (queue out=w272:refnum<queue>, error out=w274:errorcluster)  [unwired: 1 out]
        n121 = Unbundle By Name(w277) -> ("Inst_Keithley2002"=w280:refnum<queue>)
        n122 = call-poly "Enqueue Message.vi"("error in (no error)"=w274, "Message"="Leer_Frecuencia", "Message Queue"=w272) -> ("error out"=w283:errorcluster)  [unwired: 7 in, 1 out]
        n123 = call-poly "Enqueue Message.vi"("error in (no error)"=w283, "Message"="Leer_Instrumento", "Message Queue"=w280) -> ("error out"=w281:errorcluster)  [unwired: 7 in, 1 out]
        n124 = call "Time Delay2"("error in (no error)"=w281, "Delay Time (s)"=1.0) -> ("error out"=w275:errorcluster)  [unwired: 9 in]
      }
      frame "Leer_Frecuencia" {
        n125 = Flush Queue(queue=w286, error in (no error)=w289) -> (queue out=w285:refnum<queue>, error out=w287:errorcluster)  [unwired: 1 out]
        n126 = Unbundle By Name(w290) -> ("Inst_CNT90"=w293:refnum<queue>)
        n127 = call-poly "Enqueue Message.vi"("error in (no error)"=w287, "Message"="Leer_Indicadores", "Message Queue"=w285) -> ("error out"=w296:errorcluster)  [unwired: 7 in, 1 out]
        n128 = call-poly "Enqueue Message.vi"("error in (no error)"=w296, "Message"="Leer_Instrumento", "Message Queue"=w293) -> ("error out"=w294:errorcluster)  [unwired: 7 in, 1 out]
        n129 = call "Time Delay3"("error in (no error)"=w294, "Delay Time (s)"=1.0) -> ("error out"=w288:errorcluster)  [unwired: 9 in]
      }
      frame "Leer_Indicadores" {
        n130 = Flush Queue(queue=w302, error in (no error)=w308) -> (queue out=w301:refnum<queue>, error out=w303:errorcluster)  [unwired: 1 out]
        n131 = Unbundle By Name(w306) -> ("frecuencia1"=w305:refnum<vi>, "voltaje1"=w304:refnum<vi>)
        n132 = Unbundle By Name(w309) -> ("Inst_CNT90"=w312:refnum<queue>)
        n133 = property class="DigNum (strict)"(reference=w304) -> ("Value"=w298:dbl)  [unwired: 1 in, 2 out]
        "voltaje11" <- w298
        "voltaje2" <- w298
        n134 = call-poly "Enqueue Message.vi"("error in (no error)"=w303, "Message"="Leer_Voltaje", "Message Queue"=w301) -> ("error out"=w315:errorcluster)  [unwired: 7 in, 1 out]
        n135 = property class="DigNum (strict)"(reference=w305) -> ("Value"=→"frecuencia11" →"frecuencia2":dbl)  [unwired: 1 in, 2 out]
        n136 = call-poly "Enqueue Message.vi"("error in (no error)"=w315, "Message"="Leer_Instrumento", "Message Queue"=w312) -> ("error out"=w313:errorcluster)  [unwired: 7 in, 1 out]
        n137 = Bundle By Name(cluster=w306, "voltMedido"=w298) -> (w300:refnum<class "Prueba06.lvclass">)
        n138 = call "Time Delay5"("error in (no error)"=w313, "Delay Time (s)"=1.0) -> ("error out"=w307:errorcluster)  [unwired: 9 in]
      }
      frame "Detener_Instrumento" {
        w322 = "Detener_Instrumento" ("Message")
        n139 = Unbundle By Name(w318) -> ("Inst_DS360"=w325:refnum<queue>, "Inst_CNT90"=w324:refnum<queue>, "Inst_Keithley2002"=w323:refnum<queue>)
        n140 = call-poly "Enqueue Message.vi"("error in (no error)"=w319, "Message"=w322, "Message Queue"=w323) -> ("error out"=w321:errorcluster)  [unwired: 7 in, 1 out]
        n141 = call-poly "Enqueue Message.vi"("error in (no error)"=w321, "Message"=w322, "Message Queue"=w324) -> ("error out"=w320:errorcluster)  [unwired: 7 in, 1 out]
        n142 = call-poly "Enqueue Message.vi"("error in (no error)"=w320, "Message"=w322, "Message Queue"=w325) -> ("error out"=w317:errorcluster)  [unwired: 7 in, 1 out]
      }
      frame "EnviarVoltajeGEN" {
        n143 = Flush Queue(queue=w331, error in (no error)=w336) -> (queue out=w327:refnum<queue>, error out=w332:errorcluster)  [unwired: 1 out]
        n144 = Unbundle By Name(w334) -> ("Inst_DS360"=w339:refnum<queue>, "Inst_Keithley2002"=w344:refnum<queue>)
        n145 = Variant To Data(error in=w332, type=0.0, Variant=w335) -> (data=w337:dbl, error out=w342:errorcluster)
        n146 = call-poly "Enqueue Message.vi"("error in (no error)"=w342, "Message Data"=w337, "Message"="ActualizarVoltaje", "Message Queue"=w344) -> ("error out"=w340:errorcluster)  [unwired: 6 in, 1 out]
        n147 = call "Time Delay7"("error in (no error)"=w340, "Delay Time (s)"=0.5) -> ("error out"=w330:errorcluster)  [unwired: 9 in]
        n148 = local read "generar1"() -> (w326:bool)
        n149 = call-poly "Enqueue Message.vi"("error in (no error)"=w330, "Message Data"=w337, "Message"="ActualizarAmplitud", "Message Queue"=w339) -> ("error out"=w333:errorcluster)  [unwired: 6 in, 1 out]
        n150 = case shown="False" w326 {
          tunnel: w333 -> [w346 w350]
          tunnel: [w346 w349] -> w328
          tunnel: w327 -> [_ w348]
          frame False {
          }
          frame True {
            n151 = call-poly "Enqueue Message.vi"("error in (no error)"=w350, "Message"="Leer_Voltaje", "Message Queue"=w348) -> ("error out"=w349:errorcluster)  [unwired: 7 in, 1 out]
          }
        }
      }
      frame "calcularVref" {
        n152 = Unbundle By Name(w360) -> ("Tabla"=w362:string[][], "NivelSeñalRef"=w355:dbl)
        n153 = Index Array(array=w362, index (col)=1 ("disabled index (col)")) -> (element=w353:string[])  [unwired: 1 in]
        n154 = call-poly "Enqueue Message.vi"("error in (no error)"=w358, "Message"="configuraTabla", "Message Queue"=w357) -> ("error out"=w356:errorcluster)  [unwired: 7 in, 1 out]
        n155 = for {
          tunnel: w355 -> [w368]
          tunnel: [w365] -> w354 mode=indexing
          tunnel: w353 -> [w364] mode=indexing
          # "10^94/20"
          # "10^Ref/20"
          n156 = Fract/Exp String To Number(string=w364) -> (number=w374:dbl)  [unwired: 3 in, 1 out]
          n157 = Divide(x=w368, y=20.0) -> (x/y=w369:dbl)
          n158 = Divide(x=w374, y=20.0) -> (x/y=w372:dbl)
          n159 = local read "Vref"() -> (w363:dbl)
          n160 = Power Of 10(x=w369) -> (10^x=w366:dbl)
          n161 = Power Of 10(x=w372) -> (10^x=w371:dbl)
          n162 = Multiply(x=w371, y=w363) -> (x*y=w370:dbl)
          n163 = Divide(x=w370, y=w366) -> (x/y=w365:dbl)
        }
        n164 = Number To Fractional String(number=w354, precision (6)=i16 1) -> (F-format string=→"TablaVoltajes":string[])  [unwired: 2 in]
      }
      frame "configuraTabla" {
        n165 = Unbundle By Name(w388) -> ("Tabla"=w389:string[][], "Incertidumbre"=w385:string, "Tol +"=w383:string, "Tol -"=w382:string)
        n166 = local read "n° filas"() -> (w381:i32)
        n167 = call-poly "Enqueue Message.vi"("error in (no error)"=w386, "Message"="ActualizarAmplitudGEN", "Message Queue"=w376) -> ("error out"=w377:errorcluster)  [unwired: 7 in, 1 out]
        n168 = for {
          N: w381 -> [_]
          tunnel: w385 -> [w397]
          tunnel: [w397] -> w384 mode=indexing
        }
        n169 = for {
          N: w381 -> [_]
          tunnel: w383 -> [w396]
          tunnel: [w396] -> w380 mode=indexing
        }
        n170 = call "escribeEnTabla.vi"("parametros"=w384, "col"=4, "tabla in"=w389) -> ("tabla out"=w394:string[][])  [unwired: 8 in]
        n171 = for {
          N: w381 -> [_]
          tunnel: w382 -> [w395]
          tunnel: [w395] -> w379 mode=indexing
        }
        n172 = call "escribeEnTabla.vi"("parametros"=w380, "col"=5, "tabla in"=w394) -> ("tabla out"=w393:string[][])  [unwired: 8 in]
        n173 = call "escribeEnTabla.vi"("parametros"=w379, "col"=6, "tabla in"=w393) -> ("tabla out"=w378:string[][])  [unwired: 8 in]
        n174 = Bundle By Name(cluster=w388, "Tabla"=w378) -> (w387:refnum<class "Prueba06.lvclass">)
        n175 = local write "Tabla"(w378) -> ()
      }
      frame "Inicializar_Instrumento_2" {
        # "preguntamos en que valor \nde dB estamos y seleccionamos\nel voltaje a generar"
        n176 = property on="cb_rangoRef" class="CmbBox"() -> ("Value"=w414:string, "Strings[]"=w415:string[])  [unwired: 2 in, 2 out]
        n177 = local read "TablaVoltajes"() -> (w413:string[])
        n178 = Search 1D Array(1D array=w415, element=w414) -> (index of element=w398:i32)  [unwired: 1 in]
        n179 = Index Array(array=w413, index=w398) -> (element=w412:string)
        n180 = Unbundle By Name(w401) -> ("Inst_DS360"=w409:refnum<queue>, "Inst_CNT90"=w408:refnum<queue>, "Inst_Keithley2002"=w407:refnum<queue>)
        n181 = Fract/Exp String To Number(string=w412) -> (number=w411:dbl)  [unwired: 3 in, 1 out]
        n182 = local read "frecuencia1"() -> (w400:dbl)
        n183 = Divide(x=w411, y=1000.0) -> (x/y=w399:dbl)
        n184 = disable-structure shown="Enabled" {
          disable-tunnel: w416 -> [w426 w428]
          disable-tunnel: w408 -> [w425 _]
          disable-tunnel: w407 -> [w424 _]
          disable-tunnel: [w423 "Inicializar_Instrumento" ("Message")] -> w405
          disable-tunnel: [w421 w428] -> w404
          disable-tunnel: w400 -> [w420 _]
          disable-tunnel: w399 -> [w419 _]
          frame Disabled {
            w423 = "Inicializar_Instrumento" ("Message")
            n185 = call-poly "Enqueue Message.vi"("error in (no error)"=w426, "Message Data"=w419, "Message"=w423, "Message Queue"=w424) -> ("error out"=w422:errorcluster)  [unwired: 6 in, 1 out]
            n186 = call-poly "Enqueue Message.vi"("error in (no error)"=w422, "Message Data"=w420, "Message"=w423, "Message Queue"=w425) -> ("error out"=w421:errorcluster)  [unwired: 6 in, 1 out]
          }
          frame Enabled {
          }
        }
        n187 = Bundle By Name(cluster=T8 {"frec"=0.0, "amp"=0.0} ("clusterGEN"), "frec"=w400, "amp"=w399) -> (w406:T8)
        n188 = Bundle By Name(cluster=w418, "frec"=w400, "amp"=w399) -> (w417:refnum<class "Prueba06.lvclass">)
        n189 = call-poly "Enqueue Message.vi"("error in (no error)"=w404, "Message Data"=w406, "Message"=w405, "Message Queue"=w409) -> ("error out"=w402:errorcluster)  [unwired: 6 in, 1 out]
      }
      frame "ActualizarAmplitudGEN" {
        # "preguntamos en que valor \nde dB estamos y seleccionamos\nel voltaje a generar"
        n190 = property on="cb_rangoRef" class="CmbBox"() -> ("Value"=w439:string, "Strings[]"=w440:string[])  [unwired: 2 in, 2 out]
        n191 = local read "TablaVoltajes"() -> (w438:string[])
        n192 = Search 1D Array(1D array=w440, element=w439) -> (index of element=w429:i32)  [unwired: 1 in]
        "filaSelecc" <- w429
        n193 = Index Array(array=w438, index=w429) -> (element=w437:string)
        n194 = Fract/Exp String To Number(string=w437) -> (number=w436:dbl)  [unwired: 3 in, 1 out]
        n195 = Unbundle By Name(w432) -> ("Inst_DS360"=w434:refnum<queue>)
        n196 = Divide(x=w436, y=1000.0) -> (x/y=w431:dbl)
        n197 = Bundle By Name(cluster=w443, "amp"=w431) -> (w442:refnum<class "Prueba06.lvclass">)
        n198 = call-poly "Enqueue Message.vi"("error in (no error)"=w441, "Message Data"=w431, "Message"="ActualizarAmplitud", "Message Queue"=w434) -> ("error out"=w433:errorcluster)  [unwired: 6 in, 1 out]
      }
      frame "preguntaTipoPrueba" {
        n199 = Exclusive Or(1:"PruebaInf", 2:"PruebaSup") -> (0:w451:bool)
        n200 = case shown="True" w451 {
          tunnel: "PruebaSup" -> [_ w459]
          tunnel: [w457 w458] -> w447
          frame False {
            n201 = call "tipoPrueba.vi"() -> ("tipoPrueba"=w457:string)  [unwired: 1 in]
          }
          frame True {
            n202 = case shown="True" w459 {
              tunnel: ["Inferior" "Superior"] -> w458
              frame False {
              }
              frame True {
              }
            }
          }
        }
        "tipoPrueba" <- w447
        n203 = case shown="\"Superior\"" w447 {
          frame Default {
          }
          frame "Superior" {
            w454 = TRUE ("PruebaSup")
            n204 = Not(x=w454) -> (.not. x?=w453:bool)
            n205 = local write "PruebaSup"(w454) -> ()
            n206 = local write "PruebaInf"(w453) -> ()
          }
          frame "Inferior" {
            w456 = FALSE ("PruebaSup")
            n207 = Not(x=w456) -> (.not. x?=w455:bool)
            n208 = local write "PruebaSup"(w456) -> ()
            n209 = local write "PruebaInf"(w455) -> ()
          }
        }
        n210 = call-poly "Enqueue Message.vi"("error in (no error)"=w448, "Message"="iniciarGEN_2", "Message Queue"=w446) -> ("error out"=w445:errorcluster)  [unwired: 7 in, 1 out]
      }
      frame "guardarMediciones" {
        w481 = 0  # col
        # "Actualiza el nuevo valor\nde Referencia dB en Combo Box"
        # "Guarda el Valor medido en DMM\nen la Tabla"
        n211 = Unbundle By Name(w482) -> ("Tabla"=w470:string[][], "voltMedido"=w480:dbl)  [unwired: 1 out]
        n212 = Flush Queue(queue=w479, error in (no error)=w483) -> (queue out=w478:refnum<queue>, error out=w477:errorcluster)  [unwired: 1 out]
        n213 = local read "filaSelecc"() -> (w474:i32)
        n214 = Index Array(array=w470, index (col)=0 ("disabled index (col)")) -> (element=w468:string[])  [unwired: 1 in]
        n215 = call-poly "Enqueue Message.vi"("error in (no error)"=w477, "Message"="detenerGEN_2", "Message Queue"=w478) -> ("error out"=w462:errorcluster)  [unwired: 7 in, 1 out]
        n216 = call "escribeEnTablaUnValor.vi"("element"=w480, "fila"=w474, "col"=w481, "tabla in"=w470) -> ("tabla out"=w464:string[][])  [unwired: 7 in]
        n217 = Array Size(array=w468) -> (size(s)=w472:i32)
        n218 = Decrement(x=w472) -> (x-1=w471:i32)
        n219 = Greater Or Equal?(x=w474, y=w471) -> (x >= y?=w473:bool)
        n220 = Less Or Equal?(x=w474, y=0) -> (x <= y?=w467:bool)
        n221 = local read "tipoPrueba"() -> (w476:string)
        n222 = Or(x=w467, y=w473) -> (x .or. y?=w466:bool)
        n223 = Bundle By Name(cluster=w482, "Tabla"=w464) -> (w465:refnum<class "Prueba06.lvclass">)
        n224 = local write "Tabla"(w464) -> ()
        n225 = case shown="False" w466 {
          tunnel: w476 -> [w485 _]
          tunnel: w474 -> [w484 _]
          frame False {
            n226 = case shown="\"Superior\"" w485 {
              tunnel: w484 -> [w490 w492]
              tunnel: [w489 w491] -> w488
              frame "Inferior", Default {
                n227 = Increment(x=w490) -> (x+1=w489:i32)
              }
              frame "Superior" {
                n228 = Decrement(x=w492) -> (x-1=w491:i32)
              }
            }
            n229 = property on="cb_rangoRef" class="CmbBox"() -> ("Strings[]"=w487:string[])  [unwired: 2 in, 2 out]
            n230 = Index Array(array=w487, index=w488) -> (element=w486:string)
            n231 = property on="cb_rangoRef" class="CmbBox"("Value"=w486) -> ()  [unwired: 2 in, 2 out]
          }
          frame True {
            n232 = One Button Dialog(message="Llegamos al final de la Tabla") -> ()  [unwired: 1 in, 1 out]
          }
        }
      }
      frame "ingresaMediciones" {
        n233 = Flush Queue(queue=w502, error in (no error)=w508) -> (queue out=w501:refnum<queue>, error out=w503:errorcluster)  [unwired: 1 out]
        n234 = Variant To Data(error in=w503, type=string[][] [] ("NewVal"), Variant=w499) -> (data=w497:string[][], error out=w500:errorcluster)
        n235 = control-ref of="Tabla"() -> (w504:refnum<vi>)
        n236 = call "ingresaMediciones.vi"("error in (no error)"=w500, "Tbl Refnum"=w504, "New Value"=w497, "Prueba06 in"=w506) -> ("error out"=w507:errorcluster, "Prueba06 out"=w495:refnum<class "Prueba06.lvclass">)  [unwired: 6 in]
        n237 = Unbundle By Name(w495) -> ("Tabla"=w496:string[][])
        n238 = local write "Tabla"(w496) -> ()
        n239 = call-poly "Enqueue Message.vi"("error in (no error)"=w507, "Message"="cumplimiento", "Message Queue"=w501) -> ("error out"=w505:errorcluster)  [unwired: 7 in, 1 out]
      }
      frame "cumplimiento" {
        n240 = call "cumplimiento.vi"("error in (no error)"=w516, "Prueba06 in"=w514) -> ("error out"=w515:errorcluster, "Prueba06 out"=w510:refnum<class "Prueba06.lvclass">)  [unwired: 8 in]
        n241 = Unbundle By Name(w510) -> ("Tabla"=w511:string[][])
        n242 = local write "Tabla"(w511) -> ()
        n243 = call-poly "Enqueue Message.vi"("error in (no error)"=w515, "Message"="listo_evaluar", "Message Queue"=w512) -> ("error out"=w513:errorcluster)  [unwired: 7 in, 1 out]
      }
      frame "listo_evaluar" {
        n244 = Unbundle By Name(w518) -> ("Tabla"=w519:string[][])
        n245 = Index Array(array=w519, index (col)=7 ("disabled index (col)")) -> (element=w521:string[])  [unwired: 1 in]
        n246 = for {
          tunnel: [w541] -> w520 mode=indexing
          tunnel: w521 -> [w539] mode=indexing
          n247 = Not Equal?(x=w539, y="") -> (x != y?=w541:bool)
        }
        n248 = And Array Elements(Boolean array=w520) -> (logical AND=w517:bool)
        n249 = case shown="True" w517 {
          tunnel: w525 -> [w529 w538]
          tunnel: [w528 w537] -> w524
          tunnel: w523 -> [w527 w536]
          frame False {
            # "si aun no hemos temminado"
            n250 = local read "generar2"() -> (w526:bool)
            n251 = case shown="True" w526 {
              tunnel: w529 -> [w530 w534]
              tunnel: [w530 w533] -> w528
              tunnel: w527 -> [_ w532]
              frame False {
              }
              frame True {
                n252 = call-poly "Enqueue Message.vi"("error in (no error)"=w534, "Message"="Leer_Voltaje", "Message Queue"=w532) -> ("error out"=w533:errorcluster)  [unwired: 7 in, 1 out]
              }
            }
          }
          frame True {
            # "si ya se terminaron las mediciones"
            n253 = call-poly "Enqueue Message.vi"("error in (no error)"=w538, "Message"="evaluar", "Message Queue"=w536) -> ("error out"=w537:errorcluster)  [unwired: 7 in, 1 out]
          }
        }
      }
      frame "evaluar" {
        # "si todos cumplen\nentonces el ensayo\ncumple"
        n254 = Unbundle By Name(w543) -> ("Tabla"=w547:string[][])
        n255 = Index Array(array=w547, index (col)=7 ("disabled index (col)")) -> (element=w549:string[])  [unwired: 1 in]
        n256 = for {
          tunnel: [w554] -> w550 mode=indexing
          tunnel: w549 -> [w552] mode=indexing
          n257 = Equal?(x=w552, y="Cumple") -> (x = y?=w554:bool)
        }
        n258 = And Array Elements(Boolean array=w550) -> (logical AND=→"cumple_no_cumple":bool)
        n259 = call-poly "Enqueue Message.vi"("error in (no error)"=w546, "Message"="final", "Message Queue"=w545) -> ("error out"=w544:errorcluster)  [unwired: 7 in, 1 out]
      }
      frame "final" {
        n260 = local read "generar2"() -> (w555:bool)
        n261 = local read "cumple_no_cumple"() -> (w558:bool)
        "cumple" <- w558
        n262 = case shown="True" w555 {
          tunnel: w562 -> [w565 w569]
          tunnel: [w565 w568] -> w557
          tunnel: w556 -> [_ w567]
          frame False {
          }
          frame True {
            n263 = call-poly "Enqueue Message.vi"("error in (no error)"=w569, "Message"="Leer_Voltaje", "Message Queue"=w567) -> ("error out"=w568:errorcluster)  [unwired: 7 in, 1 out]
          }
        }
        n264 = Not(x=w558) -> (.not. x?=→"no_cumple":bool)
        n265 = Select(t="Cumple", s=w558, f="No Cumple") -> (s? t:f=→"resultado":string)
      }
      frame "DatoRecibidoK2002" {
        n266 = Variant To Data(error in=w573, type=0.0 ("y"), Variant=w572) -> (error out=w571:errorcluster)  [unwired: 1 out]
      }
      frame "DatoRecibidoCNT90" {
        n267 = Variant To Data(error in=w580, type=0.0, Variant=w578) -> (data=w575:dbl, error out=w579:errorcluster)
        n268 = Bundle By Name(cluster=w581, "frecMedida"=w575) -> (w576:refnum<class "Prueba06.lvclass">)
      }
      frame "detenerGEN" {
        w582 = 0.0 ("voltaje1")
        n269 = Unbundle By Name(w593) -> ("Inst_DS360"=w588:refnum<queue>)
        n270 = Flush Queue(queue=w583, error in (no error)=w592) -> (error out=w584:errorcluster)  [unwired: 2 out]
        n271 = local write "voltaje1"(w582) -> ()
        n272 = local write "voltaje2"(w582) -> ()
        n273 = local write "frecuencia1"(w582) -> ()
        n274 = local write "frecuencia2"(w582) -> ()
        n275 = call-poly "Enqueue Message.vi"("error in (no error)"=w584, "Message"="Deshabilitar_Generador", "Message Queue"=w588) -> ("error out"=w587:errorcluster)  [unwired: 7 in, 1 out]
        n276 = call "Time Delay6"("error in (no error)"=w587, "Delay Time (s)"=0.5) -> ("error out"=w586:errorcluster)  [unwired: 9 in]
        n277 = Unbundle By Name(w590) -> ("Control references"=w594:T9)
        n278 = call-poly "get control reference by name.vi"("error in (no error)"=w586, "Control name"="guardar_Vref" ("String"), "Control references"=w594) -> ("error out"=w591:errorcluster, "Ctl Refnum"=w596:refnum<vi>)  [unwired: 3 in]
        n279 = Build Array(w596) -> (w595:refnum<vi>[])
        n280 = call "Enable_Visible Buttons.vi"("Enable? (T)"=FALSE, "Controls Ref Array"=w595) -> ()  [unwired: 10 in]
      }
      frame "detenerGEN_2" {
        w618 = 0.0 ("voltaje1")
        n281 = Flush Queue(queue=w603, error in (no error)=w611) -> (queue out=w599:refnum<queue>, error out=w604:errorcluster)  [unwired: 1 out]
        n282 = Unbundle By Name(w612) -> ("Inst_DS360"=w607:refnum<queue>)
        n283 = local write "voltaje11"(w618) -> ()
        n284 = local write "voltaje2"(w618) -> ()
        n285 = local write "frecuencia1"(w618) -> ()
        n286 = local write "frecuencia2"(w618) -> ()
        n287 = call-poly "Enqueue Message.vi"("error in (no error)"=w604, "Message"="Deshabilitar_Generador", "Message Queue"=w607) -> ("error out"=w606:errorcluster)  [unwired: 7 in, 1 out]
        n288 = call "Time Delay8"("error in (no error)"=w606, "Delay Time (s)"=0.5) -> ("error out"=w601:errorcluster)  [unwired: 9 in]
        n289 = call-poly "Enqueue Message.vi"("error in (no error)"=w601, "Message"="ActualizarAmplitudGEN", "Message Queue"=w599) -> ("error out"=w600:errorcluster)  [unwired: 7 in, 1 out]
        n290 = Unbundle By Name(w609) -> ("Control references"=w613:T9)
        n291 = call-poly "get control reference by name.vi"("error in (no error)"=w600, "Control name"="guardar_Vref" ("String"), "Control references"=w613) -> ("error out"=w610:errorcluster, "Ctl Refnum"=w615:refnum<vi>)  [unwired: 3 in]
        n292 = Build Array(w615) -> (w614:refnum<vi>[])
        n293 = call "Enable_Visible Buttons.vi"("Enable? (T)"=FALSE, "Controls Ref Array"=w614) -> ()  [unwired: 10 in]
      }
      frame "guardaVerf" {
        n294 = flat-sequence {
          tunnel: w622 -> [w624]
          tunnel: [w624] -> w620
          frame #0 {
            n295 = local read "AjusteAmp"() -> (w625:T1)
            "Vref" <- w625
            n296 = Number To Fractional String(number=w625, precision (6)=i16 3) -> (F-format string=w626:string)  [unwired: 2 in]
            n297 = Format Into String(format string="Se guardó Vref = %s volts", w626) -> (resulting string=w629:string)  [unwired: 2 in, 1 out]
            n298 = One Button Dialog(message=w629) -> ()  [unwired: 1 in, 1 out]
          }
        }
        n299 = property on="seguir" class="Bool"(error in=w620, "DisabledEnum"=T4."Enabled" ("Disabled")) -> (error out=w619:errorcluster)  [unwired: 1 in, 1 out]
      }
      frame "Exit" {
        w636 = TRUE
        # "#evangelio Manda a cerrar el EHL"
        # "#evangelio Manda a cerrar todos los Loops"
        n300 = Release Queue(queue=w634, error in (no error)=w640) -> (error out=w643:errorcluster)  [unwired: 1 in, 2 out]
        n301 = Unbundle By Name(w631) -> ("Control references"=w644:T9)
        n302 = for {
          tunnel: w638 -> [w647] mode=indexing
          tunnel: w639 -> [w646]
          tunnel: TRUE -> [w645]
          n303 = call-poly "Enqueue Message.vi"("Priority Message? (F)"=w645, "Message"=w646, "Message Queue"=w647) -> ()  [unwired: 7 in, 2 out]
        }
        n304 = call "Close All Ref.vi"("error in (no error)"=w643, "Control references"=w644) -> ("error out"=w633:errorcluster)  [unwired: 9 in]
        n305 = call-dynamic "CleanUp.vi"("error in (no error)"=w633, "Prueba06 in"=w631) -> ("error out"=w632:errorcluster, "Prueba06 out"=w630:refnum<class "Prueba06.lvclass">)  [unwired: 8 in]
        n306 = call "Fire User Event - Stop.vi"("error in (no error)"=w632, "Event Data"=w636, "User Event"="Exit EHL", "User Event in"=w637) -> ("error out"=w635:errorcluster)  [unwired: 7 in]
      }
      frame "Confirmar Salida" {
        n307 = Two Button Dialog(message="¿Quieres cerrar la aplicación?", 1:"No" ("T button name (\"OK\")"), 2:"Si" ("T button name (\"OK\")")) -> (T button?=w651:bool)
        n308 = case shown="True" w651 {
          tunnel: w650 -> [w656 w658]
          tunnel: [w656 w663] -> w648
          tunnel: w649 -> [_ w659]
          frame False {
          }
          frame True {
            n309 = call-poly "Enqueue Message.vi"("error in (no error)"=w658, "Message"="Detener_Instrumento", "Message Queue"=w659) -> ("error out"=w660:errorcluster, "dup Message Queue"=w661:refnum<queue>)  [unwired: 7 in]
            n310 = call-poly "Enqueue Message.vi"("error in (no error)"=w660, "Message"="Exit", "Message Queue"=w661) -> ("error out"=w663:errorcluster)  [unwired: 7 in, 1 out]
          }
        }
      }
      frame "Error" {
        w671 = T10 1 items=["no dialog", "OK message", "continue or stop message", "OK message + warnings", "continue/stop + warnings"] ("type of dialog (OK msg:1)")
        n311 = Variant To Data(error in=w667, type=errorcluster {"status"=FALSE, "code"=0, "source"=""} ("error out"), Variant=w664) -> (data=w669:errorcluster, error out=w668:errorcluster)
        n312 = call <vilib>:"Simple Error Handler.vi"("type of dialog (OK msg:1)"=w671, "error in (no error)"=w669) -> ()  [unwired: 3 in, 5 out]
        n313 = call-poly "Enqueue Message.vi"("error in (no error)"=w668, "Message"="Exit", "Message Queue"=w666) -> ("error out"=w665:errorcluster)  [unwired: 7 in, 1 out]
      }
      frame "----------------------Controles----------------------" {
      }
      frame Default {
        n314 = xnode "Error Ring"("parameter 0"=w677) -> ("error out"=w676:errorcluster)
      }
    }
    n315 = call "Error Handler - Message Handling Loop.vi"("error in (no error)"=w96, "Message Queue"=w95) -> ("dup error in"=w93:errorcluster)  [unwired: 8 in, 1 out]
  }
  "Prueba06 out" <- w20
  n316 = call "Inst_CNT90.vi"("error in"=w3, "All Message Queues in"=w4, "Prueba31 in"=w5) -> ()  [unwired: 8 in, 1 out]
  n317 = call "Inst_DS360.vi"("error in"=w3, "All Message Queues in"=w4, "Prueba06 in"=w5) -> ()  [unwired: 8 in, 1 out]
  n318 = call "Inst_K2002.vi"("error in"=w3, "All Message Queues in"=w4, "Prueba31 in"=w5) -> ()  [unwired: 8 in, 1 out]
  n319 = Merge Errors(w19, w18) -> (→"error out":errorcluster)
